vi "initialaize.vi"(8 "error in (no error)":errorcluster, 9 "Visa com port":refnum<visa-resource-name>, 10 "Serial Device Brand":T1, 11 "Arduino in":refnum<class "Arduino.lvclass">) -> (0 "error out":errorcluster, 3 "Arduino out":refnum<class "Arduino.lvclass">)   [LabVIEW 2020, in "Arduino.lvclass"]
doc: "Override del papa Initialaize"
uses:
  Arduino.lvclass
  Combo box/serial device brand.ctl
  <vilib>/Instr/_visa.llb/VISA Configure Serial Port (Instr).vi
  Abstracts/Serial Device/Serial Device.lvclass
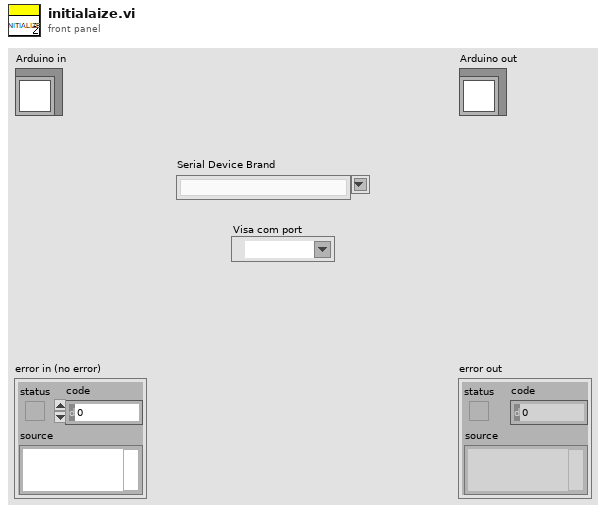
[diagram p1: front panel]
types:
  T1 = typedef "Serial Device.lvclass/serial device brand.ctl" = string
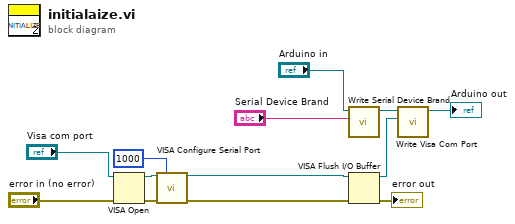
[diagram p0: block diagram]
diagram:
  n1 = VISA Open(error in (no error)="error in (no error)", VISA resource name="Visa com port") -> (VISA resource name=w13:refnum<visa-resource-name>, error out=w11:errorcluster)  [unwired: 3 in]
  n2 = call-poly "VISA Configure Serial Port"("VISA resource name"=w13, "timeout (10sec)"=u32 1000, "error in (no error)"=w11) -> ("VISA resource name out"=w2:refnum<visa-resource-name>, "error out"=w8:errorcluster)  [unwired: 11 in]
  n3 = call-dynamic "Write Serial Device Brand.vi"("Serial Device Brand"="Serial Device Brand", "Serial Device in"="Arduino in") -> ("Serial Device out"=w5:refnum<class "Arduino.lvclass">)  [unwired: 8 in, 1 out]
  n4 = VISA Flush I/O Buffer(VISA resource name=w2, error in (no error)=w8) -> (VISA resource name out=w1:refnum<visa-resource-name>, error out=→"error out":errorcluster)  [unwired: 1 in]
  n5 = call-dynamic "Write Visa Com Port.vi"("Visa Com Port"=w1, "Serial Device in"=w5) -> ("Serial Device out"=→"Arduino out":refnum<class "Arduino.lvclass">)  [unwired: 8 in, 1 out]
